vi "ImageSettings.vi"(1 "set":bool, 2 "Image Settings in":refnum<vi>) -> (0 "Image Settings out":refnum<vi>)   [LabVIEW 2009]
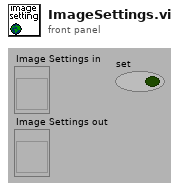
[diagram p1: front panel]
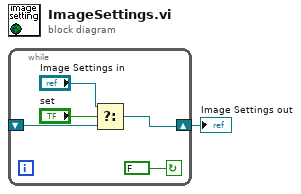
[diagram p0: block diagram]
diagram:
  n1 = while {
    shift-right: [w5] -> w1
    shift-left: _ -> [w4]
    stop <- FALSE continue-if-true
    n2 = Select(t="Image Settings in", s="set", f=w4) -> (s? t:f=w5:refnum<vi>)
  }
  "Image Settings out" <- w1
